vi "MyRio2-Camera.vi"() -> ()   [LabVIEW 2015]
uses:
  <vilib>/userdefined/High Color/IMAQdx.ctl
  <vilib>/vision/driver/NI_Vision_Acquisition_Software.lvlib
panel:
  out "Image 2":T1(plugin-control)
  out "Type":enum16{"Z", "I", "O", "S", "L", "J", "T", "N"}(ring)
  out "Discriptor":dbl[](array[numeric])
  out "Image":T1(plugin-control)
  in  "stop":bool
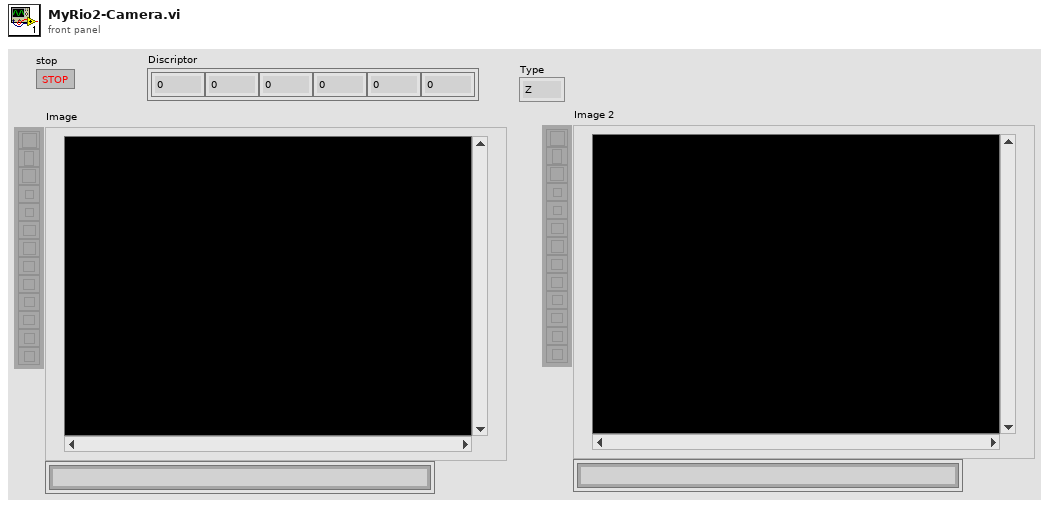
[diagram p1: front panel]
types:
  T1 = typedef "IMAQ Image.ctl" = refnum<image>
  T2 = typedef "IMAQdx.ctl" = refnum<k21>
  T3 = cluster{"p1":cluster{"x":dbl, "y":dbl}, "p2":cluster{"x":dbl, "y":dbl}}
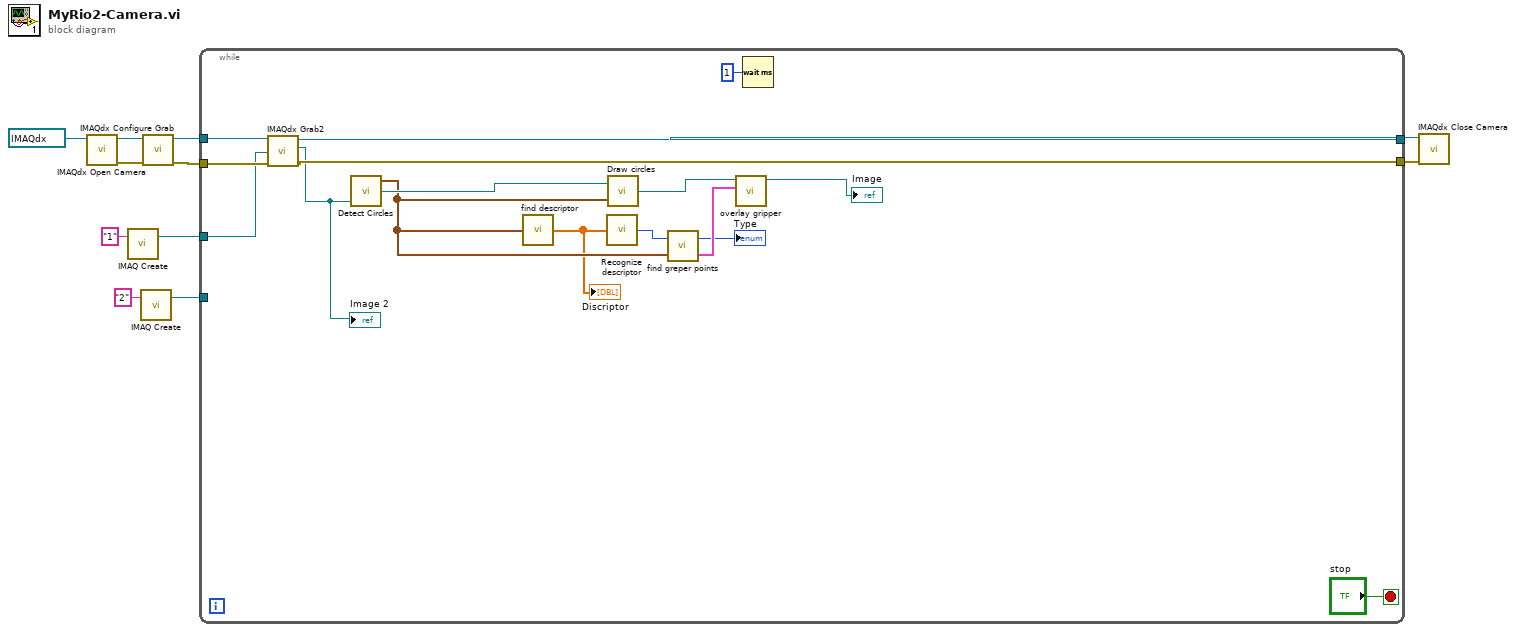
[diagram p0: block diagram]
diagram:
  n1 = call <vilib>:"IMAQdx Open Camera.vi"("Session In"=T2 "cam0") -> ("error out"=w11:errorcluster, "Session Out"=w10:T2)  [unwired: 9 in]
  n2 = call "IMAQ Create"("Image Name"="1") -> ("New Image"=w5:T1)  [unwired: 4 in, 1 out]
  n3 = call "IMAQ Create"("Image Name"="2") -> ("New Image"=w2:T1)  [unwired: 4 in, 1 out]
  n4 = call <vilib>:"IMAQdx Configure Grab.vi"("error in"=w11, "Session In"=w10) -> ("error out"=w8:errorcluster, "Session Out"=w7:T2)  [unwired: 8 in]
  n5 = while {
    tunnel: w8 -> [w27]
    tunnel: w7 -> [w26]
    tunnel: [w25] -> w6
    tunnel: w5 -> [w24]
    tunnel: w2 -> [_]
    tunnel: [w20] -> w1
    stop <- "stop" stop-if-true
    n6 = call <vilib>:"IMAQdx Grab2.vi"("error in"=w27, "Image In"=w24, "Session In"=w26) -> ("error out"=w20:errorcluster, "Image Out"=w12:T1, "Session Out"=w25:T2)  [unwired: 5 in, 1 out]
    "Image 2" <- w12
    n7 = call "Detect Circles.vi"("Image"=w12) -> ("Image 2"=w21:T1, "Circles"=w19:cluster{"x":dbl, "y":dbl, "r":dbl}[])  [unwired: 2 in, 1 out]
    n8 = call "find descriptor.vi"("Circles"=w19) -> ("d"=w13:dbl[])
    "Discriptor" <- w13
    n9 = call "Recognize descriptor.vi"("Discriptor"=w13) -> ("Type"=w16:enum16{"Z", "I", "O", "S", "L", "J", "T", "N"})
    n10 = call "Draw circles .vi"("Circles"=w19, "Refnum in"=w21) -> ("Refnum out"=w18:T1)
    n11 = call "find greper points.vi"("Circles"=w19, "Type  2"=w16) -> ("gripper"=w17:T3, "Type"=→"Type":enum16{"Z", "I", "O", "S", "L", "J", "T", "N"})
    n12 = call "overlay gripper.vi"("gripper"=w17, "Refnum in"=w18) -> ("Refnum out"=→"Image":T1)  [unwired: 9 in]
    n13 = Wait (ms)(milliseconds to wait=u32 1) -> ()  [unwired: 1 out]
  }
  n14 = call <vilib>:"IMAQdx Close Camera.vi"("error in"=w1, "Session In"=w6) -> ()  [unwired: 9 in, 1 out]
